vi "1-地址-账户信息-html - 副本.vi"(8 "error in (no error)":errorcluster caption="错误输入（无错误）", 11 "URL输入":string="https://chain.api.btc.com/v3/address/15urYnyeJe3gwbGJ74wcX89Tz7ZtsFDVew/tx") -> (0 "error out":errorcluster caption="错误输出", 1 "headers":string caption="头部", 2 "body":string caption="体部", 3 "URL输出":string)   [LabVIEW 2020]
uses:
  <vilib>/httpClient/ClientHandle.ctl
  <vilib>/httpClient/LabVIEWHTTPClient.lvlib
panel:
  in  "client handle":T1 caption="客户端句柄"
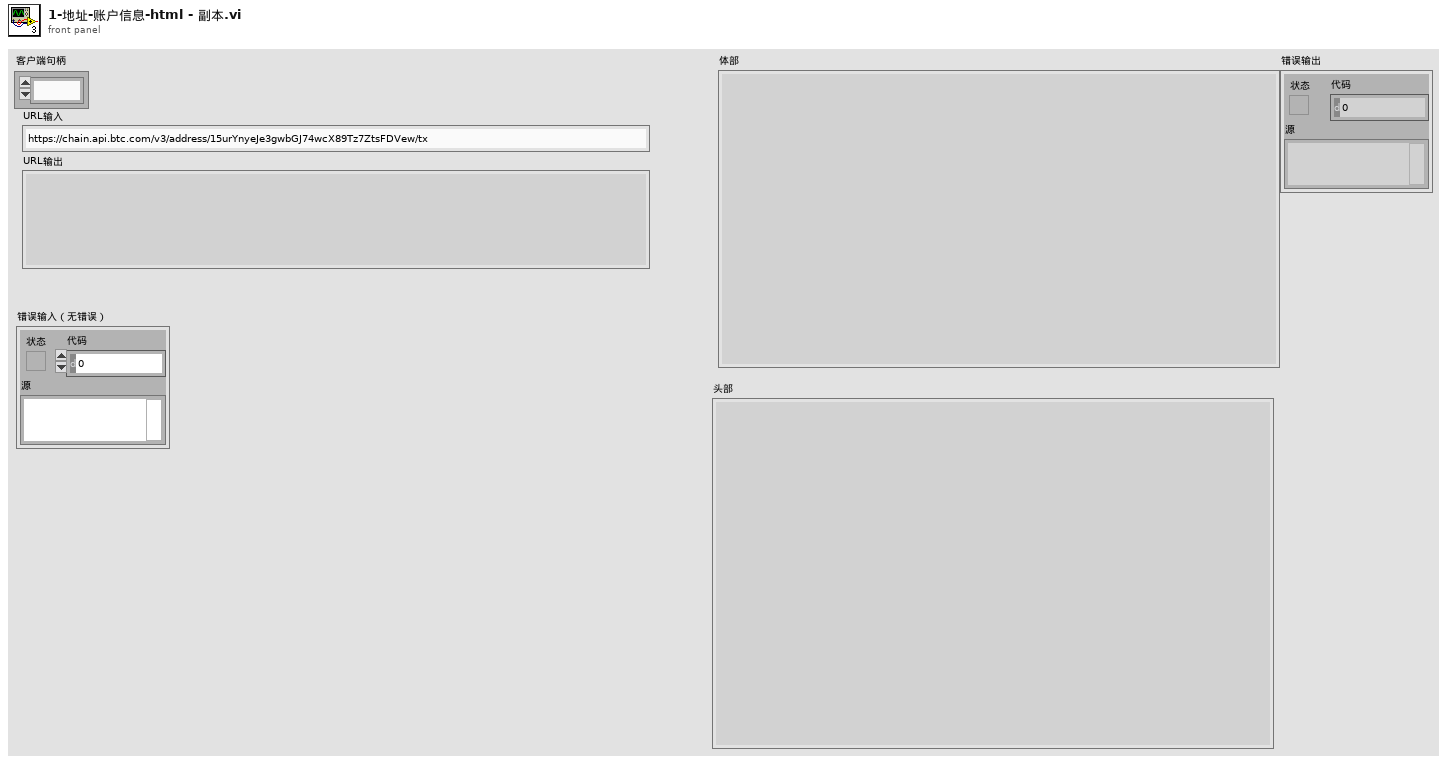
[diagram p1: front panel]
types:
  T1 = typedef "LabVIEWHTTPClient.lvlib/ClientHandle.ctl" = refnum<k1>
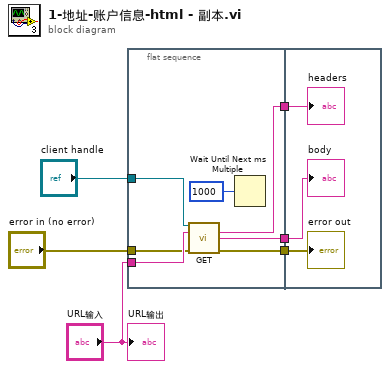
[diagram p0: block diagram]
diagram:
  n1 = flat-sequence {
    tunnel: [w10] -> w6
    tunnel: [w9] -> w5
    tunnel: "client handle" -> [w13]
    tunnel: "URL输入" -> [w12]
    tunnel: "error in (no error)" -> [w11]
    tunnel: [w7] -> w4
    tunnel: w6 -> [w16]
    tunnel: w5 -> [w15]
    tunnel: w4 -> [w14]
    frame #0 {
      n2 = call <vilib>:"GET.vi"("client handle"=w13, "url"=w12, "error in (no error)"=w11) -> ("headers"=w10:string, "body"=w9:string, "error out"=w7:errorcluster)  [unwired: 9 in, 1 out]
      n3 = Wait Until Next ms Multiple(millisecond multiple=u32 1000 ("毫秒倍数")) -> ()  [unwired: 1 out]
    }
    frame #1 {
      "body" <- w15
      "headers" <- w16
      "error out" <- w14
    }
  }
  "URL输出" <- "URL输入"
